vi "RegisterWriteTest (FPGA).vi"() -> ()   [LabVIEW 2012]
uses:
  <vilib>/eio/EIONode/EIONode.xnode
panel:
  in  "Count(uSec)":u32=800
  in  "Point":cluster{"X":i32, "Y":i32, "Z":i32} {"Z" format="%x"; "Y" format="%x"; "X" format="%x"}
  in  "UpdatesPerPoint":u32
  in  "stop 2":bool
  in  "Write Points":bool
  in  "P":bool
  in  "stop":bool
  in  "Pause":u32
  in  "WriteSize":enum16{"1", "2", "4"}(ring)
  in  "Divider":u32=2
  in  "NumRegs":i16=10
  in  "Update IO time":u32=20
  in  "Register  Values":cluster{"Address":u8, "Value":u32}[](array[cluster])=[{"Address"=0, "Value"=240}, {"Address"=1, "Value"=13762592}, {"Address"=2, "Value"=32768}, {"Address"=3, "Value"=8413952}, {"Address"=4, "Value"=858993459}, {"Address"=5, "Value"=0}, {"Address"=6, "Value"=1023}, {"Address"=7, "Value"=257}, {"Address"=8, "Value"=21}, {"Address"=10, "Value"=858993459}, {"Address"=0, "Value"=240}, {"Address"=0, "Value"=0}, {"Address"=0, "Value"=0}, {"Address"=0, "Value"=0}, {"Address"=0, "Value"=0}, {"Address"=0, "Value"=0}, {"Address"=0, "Value"=0}, {"Address"=0, "Value"=0}, {"Address"=0, "Value"=0}, {"Address"=0, "Value"=0}] {"Address" format="%x"; "Value" format="%x"}
  in  "Write Registers":bool
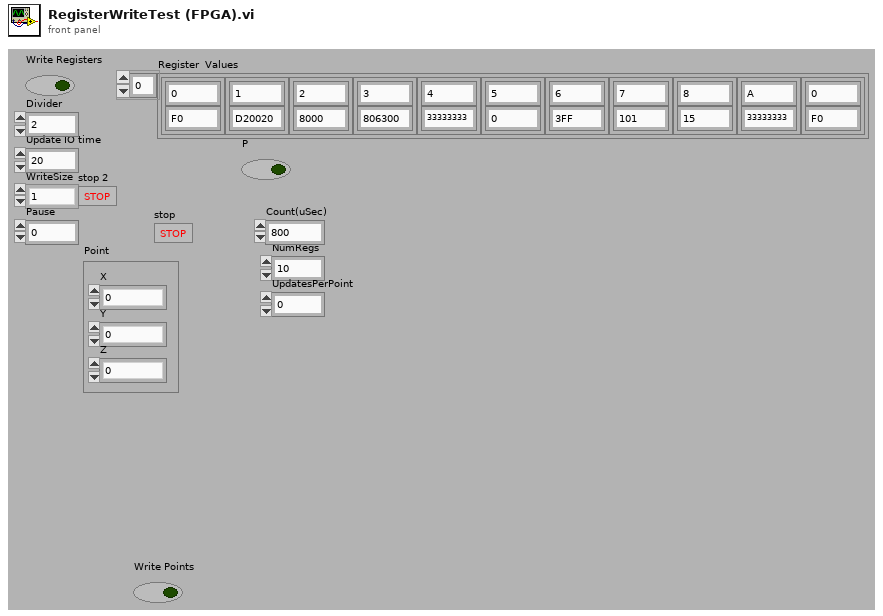
[diagram p1: front panel]
types:
  T1 = typedef "CoordinateSettings.ctl" = cluster{"XHPstart":u32, "XHPend":u32, "XLPstart":u32, "XLPend":u32, "YHPstart":u32, "YHPend":u32, "YLPstart":u32, "YLPend":u32, "XHP_RR":u32, "XHP_FR":u32, "XLP_FR":u32, "XLP_RR":u32, "YHP_FR":u32, "YHP_RR":u32, "YLP_FR":u32, "YLP_RR":u32}
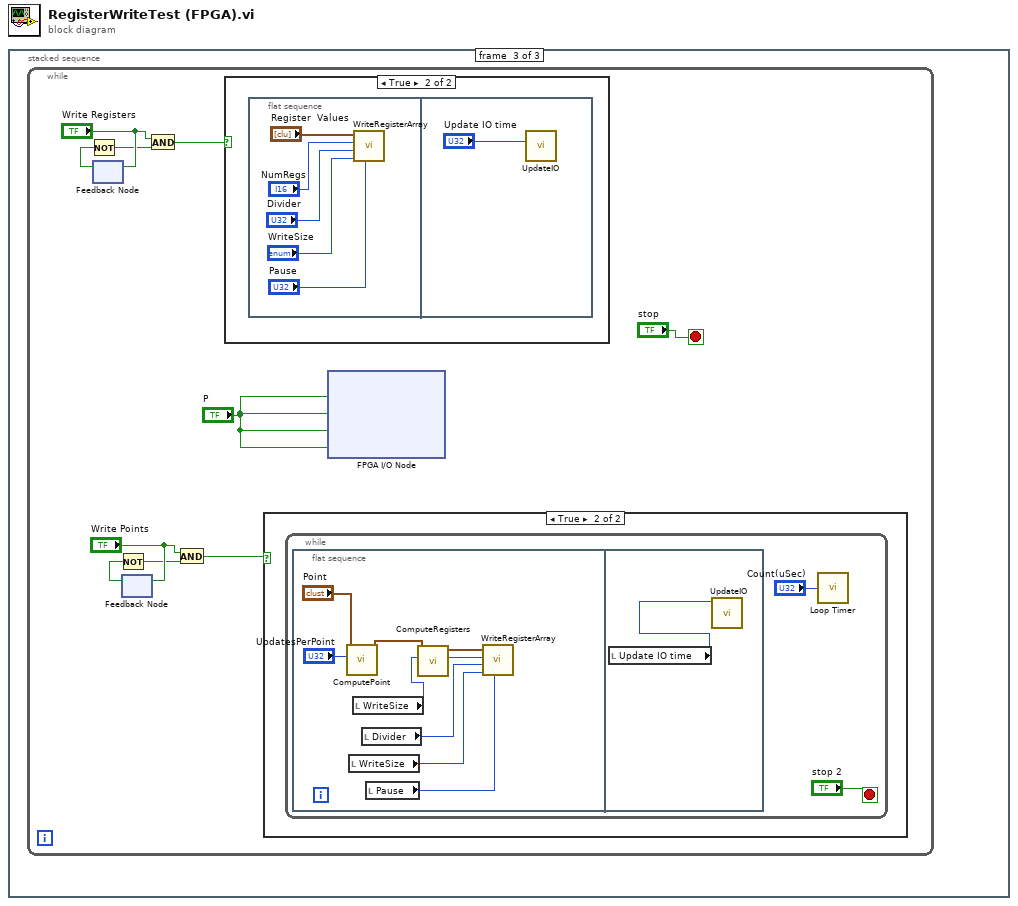
[diagram p0: block diagram]
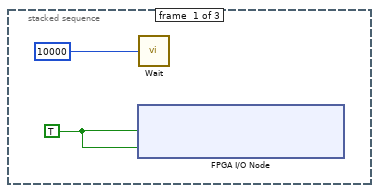
[diagram p2: hidden frame]
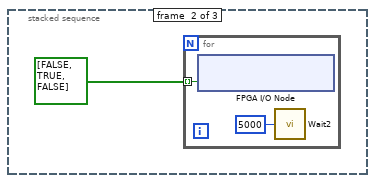
[diagram p3: hidden frame]
diagram:
  n1 = stacked-sequence {
    frame #0 {
      w1 = TRUE ("IO Module\\DDCA_DIO0-7_WE")
      n2 = xnode "FPGA I/O Node"("IO Module\\DDCA_DIO0-7_WE"=w1, "IO Module\\DDCA_DIO8-15_WE"=w1) -> ()  [unwired: 2 in, 2 out]
      n3 = call "Wait"("Count(uSec)"=u32 10000) -> ()  [unwired: 1 out]
    }
    frame #1 {
      n4 = for {
        tunnel: bool[] [FALSE, TRUE, FALSE] -> [w4] mode=indexing
        n5 = xnode "FPGA I/O Node"("IO Module\\RESET"=w4) -> ()  [unwired: 1 in, 1 out]
        n6 = call "Wait2"("Count(uSec)"=u32 5000) -> ()  [unwired: 1 out]
      }
    }
    frame #2 {
      n7 = while {
        stop <- "stop" stop-if-true
        n8 = feedback-in #1("Write Registers") -> ()
        n9 = feedback #1() -> (w15:bool)  [unwired: 1 in]
        n10 = Not(x=w15) -> (.not. x?=w13:bool)
        n11 = feedback-in #2("Write Points") -> ()
        n12 = feedback #2() -> (w9:bool)  [unwired: 1 in]
        n13 = Not(x=w9) -> (.not. x?=w7:bool)
        n14 = And(x="Write Registers", y=w13) -> (x .and. y?=w12:bool)
        n15 = And(x="Write Points", y=w7) -> (x .and. y?=w6:bool)
        n16 = case shown="True" w12 {
          frame False {
          }
          frame True {
            n17 = flat-sequence {
              frame #0 {
                n18 = call "WriteRegisterArray.vi"("Pause"="Pause", "WriteSize"="WriteSize", "SclkDivider"="Divider", "NumReg"="NumRegs", "Register  Values"="Register  Values") -> ()  [unwired: 7 in]
              }
              frame #1 {
                n19 = call "UpdateIO.vi"("Count(ticks)"="Update IO time") -> ()  [unwired: 11 in]
              }
            }
          }
        }
        n20 = case shown="True" w6 {
          frame False {
          }
          frame True {
            n21 = while {
              stop <- "stop 2" stop-if-true
              n22 = flat-sequence {
                frame #0 {
                  n23 = call "ComputePoint.vi"("UpdatesPerPoint"="UpdatesPerPoint", "Point"="Point") -> ("settings"=w26:T1)  [unwired: 9 in]
                  n24 = local read "WriteSize"() -> (w22:enum16{"1", "2", "4"})
                  n25 = local read "WriteSize"() -> (w25:enum16{"1", "2", "4"})
                  n26 = local read "Divider"() -> (w21:u32)
                  n27 = local read "Pause"() -> (w20:u32)
                  n28 = call "ComputeRegisters.vi"("WriteSize"=w25, "coordinates"=w26) -> ("Numeric"=w23:i16, "Register Writes"=w24:cluster{"Address":u8, "Value":u32}[])  [unwired: 8 in]
                  n29 = call "WriteRegisterArray.vi"("Pause"=w20, "WriteSize"=w22, "SclkDivider"=w21, "NumReg"=w23, "Register  Values"=w24) -> ()  [unwired: 7 in]
                }
                frame #1 {
                  n30 = local read "Update IO time"() -> (w27:u32)
                  n31 = call "UpdateIO.vi"("Count(ticks)"=w27) -> ()  [unwired: 11 in]
                }
              }
              n32 = call "Loop Timer"("Count(uSec)"="Count(uSec)") -> ()  [unwired: 1 out]
            }
          }
        }
        n33 = xnode "FPGA I/O Node"("IO Module\\P0"="P", "IO Module\\P1"="P", "IO Module\\P2"="P", "IO Module\\P3"="P") -> ()  [unwired: 4 in, 4 out]
      }
    }
  }
